vi "PruebaDAQ_ElminMejia_LesterRoche.vi"() -> ()   [LabVIEW 2011]
panel:
  in  "stop":bool
  out "Alarma de temp.":bool
  out "Temperatura":i32(knob) scale=0.0..5.0
  out "Encendido":bool
  out "Cuarta":bool
  out "Tercera":bool
  out "Segunda":bool
  out "Primera":bool
  out "Brake":bool
  out "Acelerador":bool
  out "velocidad":i32(knob) scale=1.0..220.0
  # "Se tiene que generar la temperatura del auto de acuerdo\na la velocidad:\n1-70 temp 1-2\n70-130 temp 1-4\n130- temp 1-5\nEsto es una entrada  que se escribe en la temperatura\ny salida analogica que se ingresa del valor de la temperatura\na la daq.\n\nEl acelerador cada vez que se pulsa el boton que sera \nuna entrada de la daq aumenta la velocidad en 10.\nSi se presiona el boton del brake se rebaja la velocidad.\n\nDebera de producirse 4 salidas digitales para representar \ncada uno de los cambios usando led\n1-30 primera\n31-50 segunda\n50-80 tercera\n80- cuarta\n\nLa alarma de la temperatura se enciende solo si esta\nsube de 3 enciende un led en la daq, la que es una \nsalida digital."
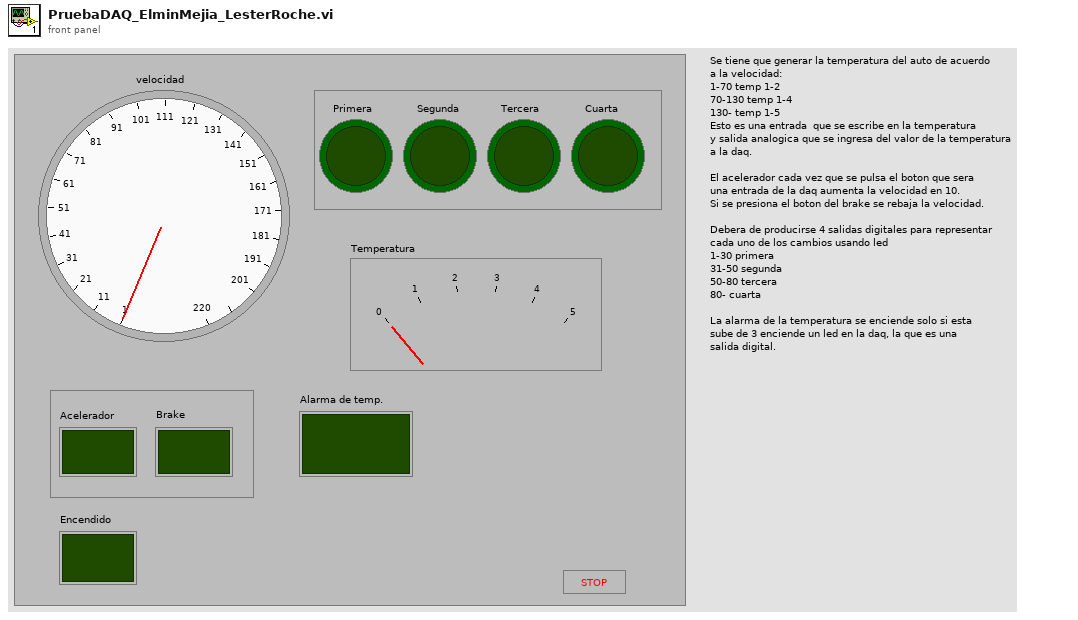
[diagram p1: front panel]
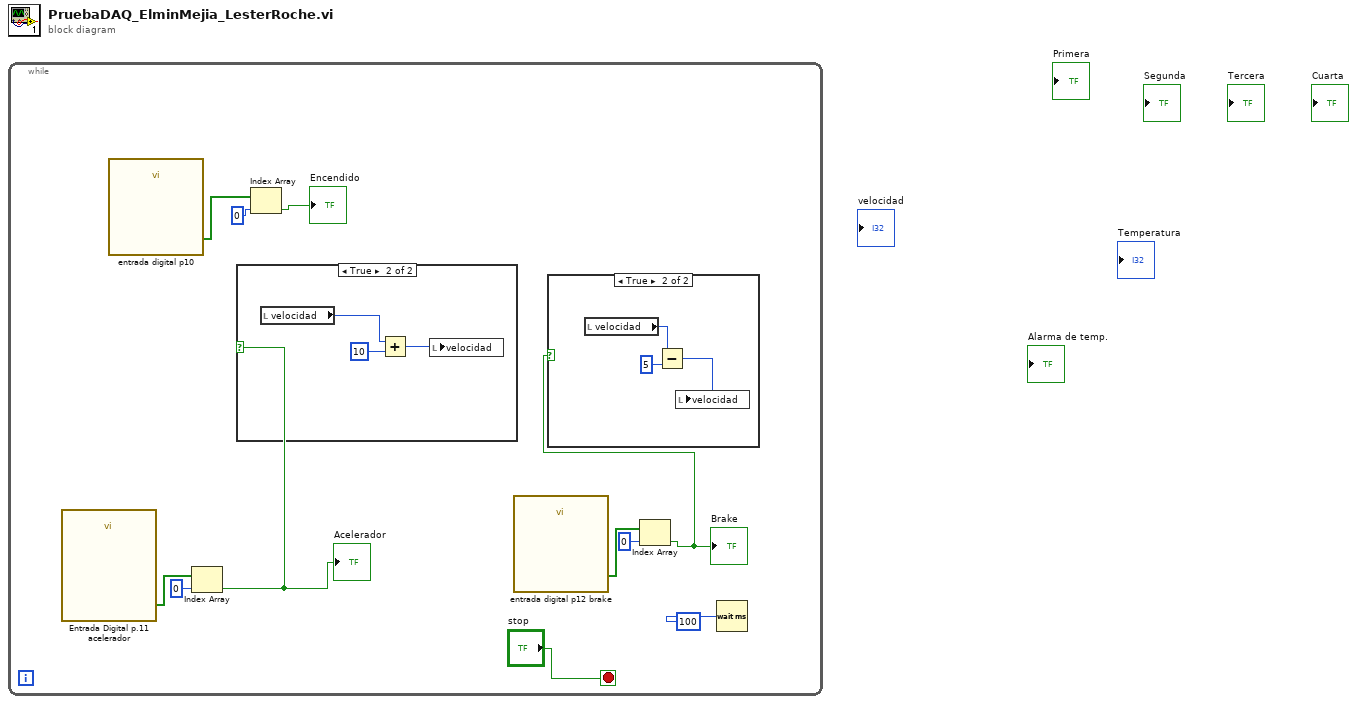
[diagram p0: block diagram]
diagram:
  n1 = while {
    stop <- "stop" stop-if-true
    n2 = call "Entrada Digital p.11 acelerador"() -> ("data"=w7:bool[])  [unwired: 17 in, 2 out]
    n3 = call "entrada digital p10"() -> ("data"=w10:bool[])  [unwired: 17 in, 2 out]
    n4 = Index Array(array=w7, index=0) -> (element=w5:bool)
    "Acelerador" <- w5
    n5 = case shown="True" w5 {
      frame False {
      }
      frame True {
        n6 = local read "velocidad"() -> (w16:i32)
        n7 = Add(x=w16, y=10) -> (x+y=w15:i32)
        n8 = local write "velocidad"(w15) -> ()
      }
    }
    n9 = Index Array(array=w10, index=0) -> (element=→"Encendido":bool)
    n10 = call "entrada digital p12 brake"() -> ("data"=w3:bool[])  [unwired: 17 in, 2 out]
    n11 = Index Array(array=w3, index=0) -> (element=w1:bool)
    "Brake" <- w1
    n12 = case shown="True" w1 {
      frame False {
      }
      frame True {
        n13 = local read "velocidad"() -> (w13:i32)
        n14 = Subtract(x=w13, y=5) -> (x-y=w12:i32)
        n15 = local write "velocidad"(w12) -> ()
      }
    }
    n16 = Wait (ms)(milliseconds to wait=u32 100) -> ()  [unwired: 1 out]
  }
